vi "MGCC_FntStaMach_Error_State_Control_main.vi"() -> ()   [LabVIEW 2016]
doc: "-----------------------------------------------------------------------------------------------------------------------\nCopyright <2019> <The University of Tennessee at Knoxville and the University of Tennessee Research Foundation>\nThis software is released under BSD-3 \nhttps://opensource.org/licenses/BSD-3-Clause \nAdditional license options available at https://utrf.tennessee.edu/industry/sample-agreements/\n-----------------------------------------------------------------------------------------------------------------------"
uses:
  Sub_VIs/Fault_Abnormal_state.vi
panel:
  out "appended array":errorcluster[](array[cluster])
  in  "Boolean 2":bool
  out "Boolean":bool
  out "result":bool
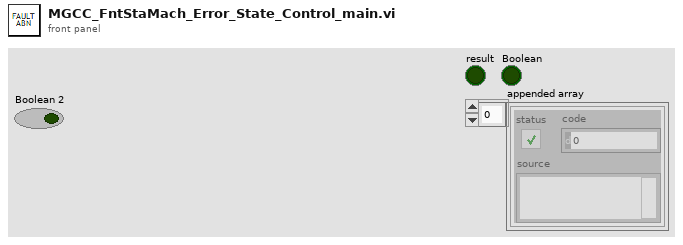
[diagram p1: front panel]
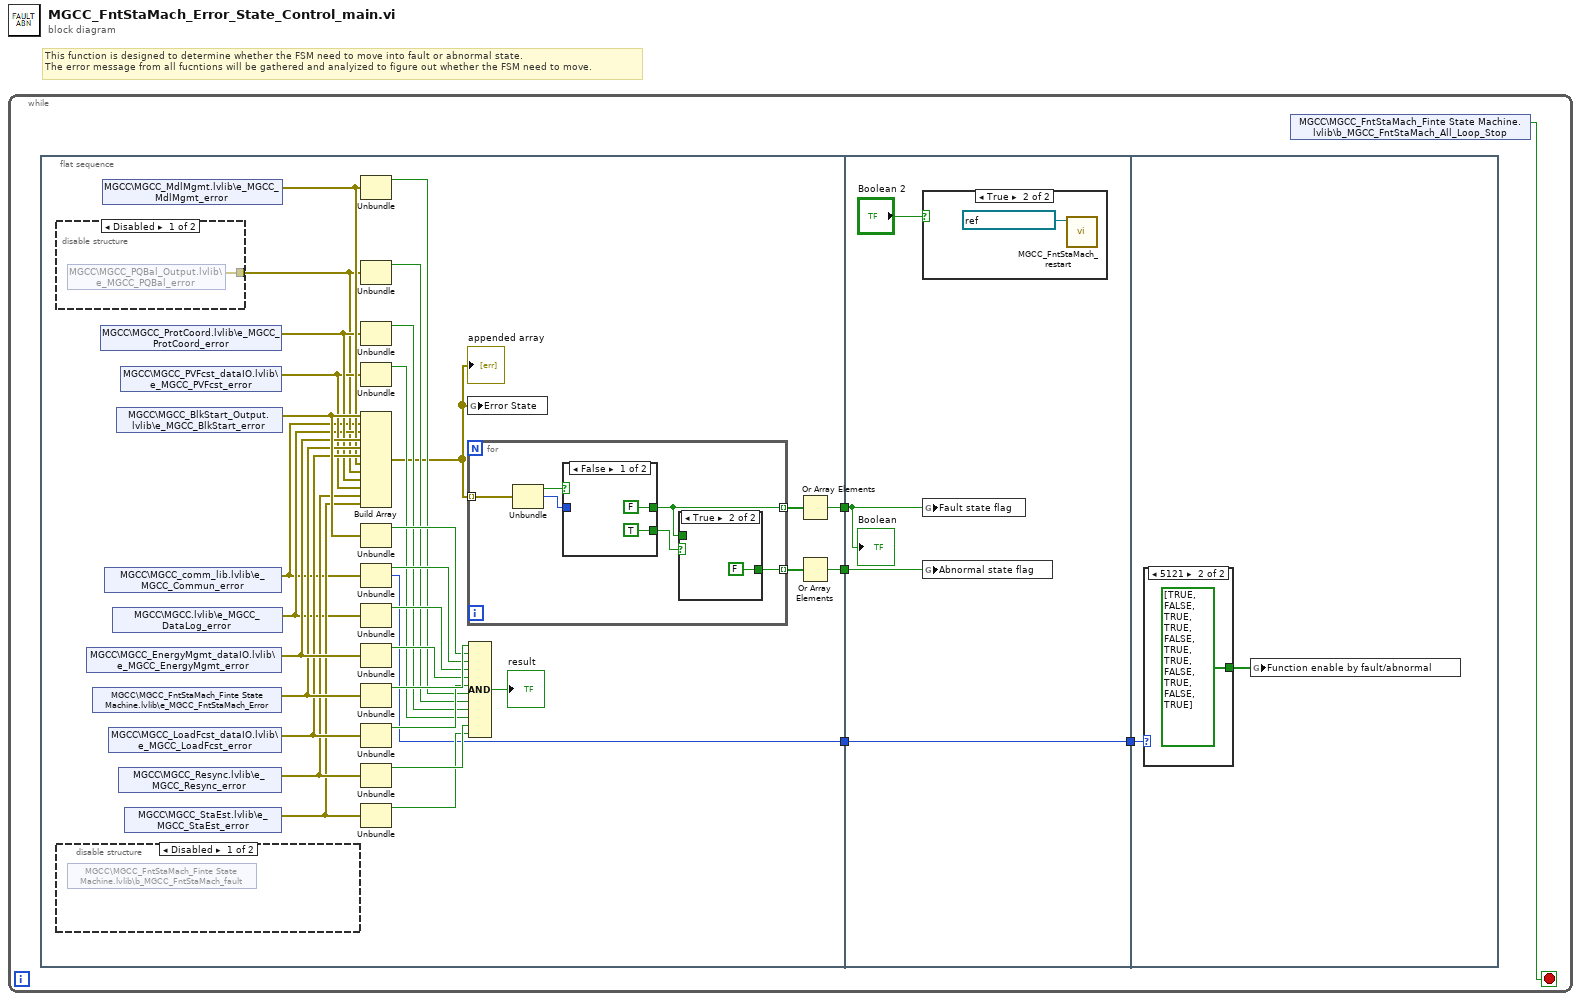
[diagram p0: block diagram]
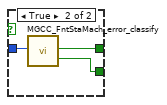
[diagram p3: hidden frame]
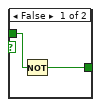
[diagram p4: hidden frame]
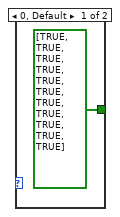
[diagram p7: hidden frame]
diagram:
  # "This function is designed to determine whether the FSM need to move into fault or abnormal state.\nThe error message from all fucntions will be gathered and analyized to figure out whether the FSM need to move."
  n1 = while {
    stop <- w5 stop-if-true
    n2 = flat-sequence {
      tunnel: [w10] -> w4
      tunnel: [w11] -> w3
      tunnel: [w6] -> w1
      tunnel: w4 -> [w54]
      tunnel: w3 -> [w53]
      tunnel: [w52] -> w2
      tunnel: w1 -> [w52]
      tunnel: w2 -> [w58]
      frame #0 {
        n3 = disable-structure shown="Disabled" {
          disable-tunnel: [w37 _] -> w9
          frame Disabled {
            n4 = shared-variable "MGCC\\MGCC_PQBal_Output.lvlib\\e_MGCC_PQBal_error"() -> (w37:errorcluster)  [unwired: 1 in, 1 out]
          }
          frame Enabled {
          }
        }
        n5 = disable-structure shown="Disabled" {
          frame Disabled {
            n6 = shared-variable "MGCC\\MGCC_FntStaMach_Finte State Machine.lvlib\\b_MGCC_FntStaMach_fault"() -> ()  [unwired: 2 in, 1 out]
          }
          frame Enabled {
          }
        }
        n7 = shared-variable "MGCC\\MGCC_EnergyMgmt_dataIO.lvlib\\e_MGCC_EnergyMgmt_error"() -> (w22:errorcluster)  [unwired: 1 in, 1 out]
        n8 = shared-variable "MGCC\\MGCC_FntStaMach_Finte State Machine.lvlib\\e_MGCC_FntStaMach_Error"() -> (w21:errorcluster)  [unwired: 1 in, 1 out]
        n9 = shared-variable "MGCC\\MGCC_ProtCoord.lvlib\\e_MGCC_ProtCoord_error"() -> (w18:errorcluster)  [unwired: 1 in, 1 out]
        n10 = shared-variable "MGCC\\MGCC_MdlMgmt.lvlib\\e_MGCC_MdlMgmt_error"() -> (w19:errorcluster)  [unwired: 1 in, 1 out]
        n11 = shared-variable "MGCC\\MGCC_comm_lib.lvlib\\e_MGCC_Commun_error"() -> (w8:errorcluster)  [unwired: 1 in, 1 out]
        n12 = shared-variable "MGCC\\MGCC_LoadFcst_dataIO.lvlib\\e_MGCC_LoadFcst_error"() -> (w20:errorcluster)  [unwired: 1 in, 1 out]
        n13 = shared-variable "MGCC\\MGCC.lvlib\\e_MGCC_DataLog_error"() -> (w14:errorcluster)  [unwired: 1 in, 1 out]
        n14 = shared-variable "MGCC\\MGCC_BlkStart_Output.lvlib\\e_MGCC_BlkStart_error"() -> (w23:errorcluster)  [unwired: 1 in, 1 out]
        n15 = shared-variable "MGCC\\MGCC_Resync.lvlib\\e_MGCC_Resync_error"() -> (w16:errorcluster)  [unwired: 1 in, 1 out]
        n16 = shared-variable "MGCC\\MGCC_PVFcst_dataIO.lvlib\\e_MGCC_PVFcst_error"() -> (w17:errorcluster)  [unwired: 1 in, 1 out]
        n17 = shared-variable "MGCC\\MGCC_StaEst.lvlib\\e_MGCC_StaEst_error"() -> (w15:errorcluster)  [unwired: 1 in, 1 out]
        n18 = Unbundle(w19) -> ("status"=w30:bool)  [unwired: 2 out]
        n19 = Unbundle(w9) -> ("status"=w29:bool)  [unwired: 2 out]
        n20 = Unbundle(w18) -> ("status"=w28:bool)  [unwired: 2 out]
        n21 = Unbundle(w17) -> ("status"=w27:bool)  [unwired: 2 out]
        n22 = Build Array(w23, w8, w14, w22, w21, w20, w19, w9, w18, w17, w16, w15) -> (w7:errorcluster[])
        "appended array" <- w7
        n23 = Unbundle(w23) -> ("status"=w35:bool)  [unwired: 2 out]
        n24 = Unbundle(w8) -> ("status"=w34:bool, "code"=w6:i32)  [unwired: 1 out]
        n25 = Unbundle(w14) -> ("status"=w33:bool)  [unwired: 2 out]
        n26 = Unbundle(w22) -> ("status"=w32:bool)  [unwired: 2 out]
        n27 = Unbundle(w21) -> ("status"=w36:bool)  [unwired: 2 out]
        n28 = Unbundle(w20) -> ("status"=w31:bool)  [unwired: 2 out]
        n29 = Unbundle(w16) -> ("status"=w26:bool)  [unwired: 2 out]
        n30 = Unbundle(w15) -> ("status"=w25:bool)  [unwired: 2 out]
        n31 = global write "Fault_Abnormal_state.vi" "Error State"(w7) -> ()
        n32 = for {
          tunnel: w7 -> [w41] mode=indexing
          tunnel: [w40] -> w13 mode=indexing
          tunnel: [w39] -> w12 mode=indexing
          n33 = Unbundle(w41) -> ("status"=w38:bool, "code"=w43:i32)  [unwired: 1 out]
          n34 = case shown="False" w38 {
            tunnel: w43 -> [_ w48]
            tunnel: [TRUE ("No error") w47] -> w42
            tunnel: [FALSE ("Error state") w46] -> w40
            frame False {
            }
            frame True {
              n35 = call "MGCC_FntStaMach_error_classify.vi"("Error"=w48) -> ("Error state"=w46:bool, "No error"=w47:bool)  [unwired: 17 in]
            }
          }
          n36 = case shown="True" w42 {
            tunnel: [w49 FALSE] -> w39
            tunnel: w40 -> [w50 _]
            frame False {
              n37 = Not(x=w50) -> (.not. x?=w49:bool)
            }
            frame True {
            }
          }
        }
        n38 = Compound Arithmetic op=AND(w36, w35, w34, w33, w32, w31, w30, w29, w28, w27, w26, w25) -> (→"result":bool)
        n39 = Or Array Elements(Boolean array=w13) -> (logical OR=w10:bool)
        n40 = Or Array Elements(Boolean array=w12) -> (logical OR=w11:bool)
      }
      frame #1 {
        n41 = case shown="True" "Boolean 2" {
          frame False {
          }
          frame True {
            n42 = call "MGCC_FntStaMach_restart.vi"("Session in"=refnum<k21> "48.26.87.212") -> ()  [unwired: 8 in, 3 out]
          }
        }
        n43 = global write "Fault_Abnormal_state.vi" "Fault state flag"(w54) -> ()
        n44 = global write "Fault_Abnormal_state.vi" "Abnormal state flag"(w53) -> ()
        "Boolean" <- w54
      }
      frame #2 {
        n45 = case shown="5121" w58 {
          tunnel: [bool[] [TRUE, TRUE, TRUE, TRUE, TRUE, TRUE, TRUE, TRUE, TRUE, TRUE, TRUE] ("Function enable by fault/abnormal") bool[] [TRUE, FALSE, TRUE, TRUE, FALSE, TRUE, TRUE, FALSE, TRUE, FALSE, TRUE] ("Function enable by fault/abnormal")] -> w57
          frame 0, Default {
          }
          frame 5121 {
          }
        }
        n46 = global write "Fault_Abnormal_state.vi" "Function enable by fault/abnormal"(w57) -> ()
      }
    }
    n47 = shared-variable "MGCC\\MGCC_FntStaMach_Finte State Machine.lvlib\\b_MGCC_FntStaMach_All_Loop_Stop"() -> (w5:bool)  [unwired: 1 in, 1 out]
  }
